vi "Get Ring Exposure Range.vi"(8 "error in (no error)":errorcluster, 10 "fpMax":sgl, 11 "fpMin":sgl) -> (0 "error out":errorcluster, 1 "function return":u32, 2 "fpMax out":sgl, 3 "fpMin out":sgl)   [LabVIEW 2014, in "atmcd32d.lvlib"]
doc: "unsigned int WINAPI GetRingExposureRange(float * fpMin, float * fpMax);"
uses:
  atmcd32d.lvlib
  atmcd32d.dll
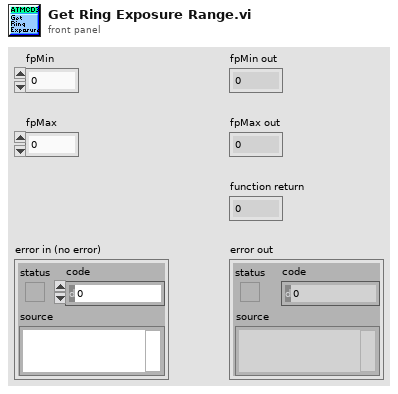
[diagram p1: front panel]
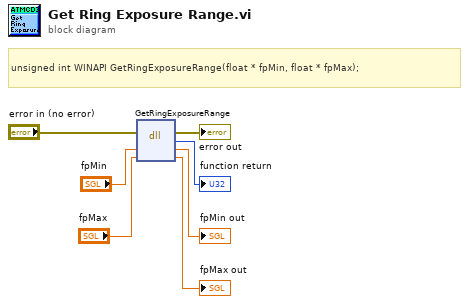
[diagram p0: block diagram]
diagram:
  # "unsigned int WINAPI GetRingExposureRange(float * fpMin, float * fpMax);"
  n1 = dll-call lib="C:/Users/Bakir/Documents/Lambda2-Testing/lib/Andorlib/atmcd32d.*" fn="GetRingExposureRange"(error in="error in (no error)", "fpMin"="fpMin", "fpMax"="fpMax") -> (error out=→"error out":errorcluster, →"function return":u32, "fpMin"=→"fpMin out":sgl, "fpMax"=→"fpMax out":sgl)  [unwired: 2 in, 1 out]
